vi "LoadApplicationConfig.vi"(8 "error in (no error)":errorcluster) -> (0 "error out":errorcluster, 2 "Config Cluster":T1, 3 "refnum out":T7)   [LabVIEW 2026]
uses:
  <vilib>/Utility/config.llb/Config Data RefNum.ctl
  Controls/Vibration_Monitor_Config.ctl
  Controls/Vibration_Profile.ctl
  Controls/System_Settings.ctl
  Controls/Options.ctl
  Controls/Relay_Profile.ctl
  Controls/RPM_Profile.ctl
  <vilib>/Utility/config.llb/Read Key (String).vi
  <vilib>/Utility/config.llb/Read Key (I32).vi
  <vilib>/Utility/config.llb/Read Key (Double).vi
  <vilib>/Utility/config.llb/NI_LVConfig.lvlib
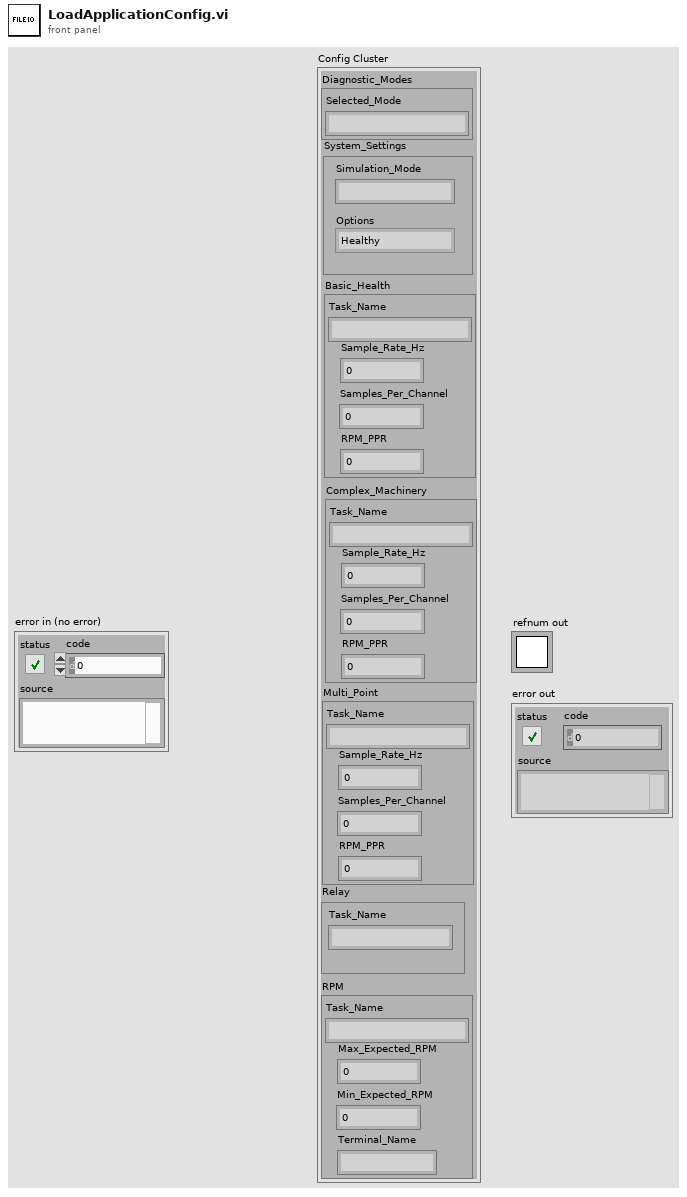
[diagram p1: front panel]
types:
  T1 = typedef "Vibration_Monitor_Config.ctl" = cluster{"Diagnostic_Modes":cluster{"Selected_Mode":string}, "Basic_Health":T2, "Complex_Machinery":T2, "Multi_Point":T2, "System_Settings":T3, "Relay":T5, "RPM":T6}
  T2 = typedef "Vibration_Profile.ctl" = cluster{"Task_Name":string, "Sample_Rate_Hz":dbl, "Samples_Per_Channel":i32, "RPM_PPR ":dbl}
  T3 = typedef "System_Settings.ctl" = cluster{"Simulation_Mode ":string, "Options":T4}
  T4 = typedef "Options.ctl" = enum16{"Healthy", "Unbalance_Alert", "Bearing_Fault_Critical", "Sweep_Test"}
  T5 = typedef "Relay_Profile.ctl" = cluster{"Task_Name":string}
  T6 = typedef "RPM_Profile.ctl" = cluster{"Task_Name":string, "Max_Expected_RPM":dbl, "Min_Expected_RPM":dbl, "Terminal_Name":string}
  T7 = typedef "NI_LVConfig.lvlib/Config Data RefNum.ctl" = refnum<k1>
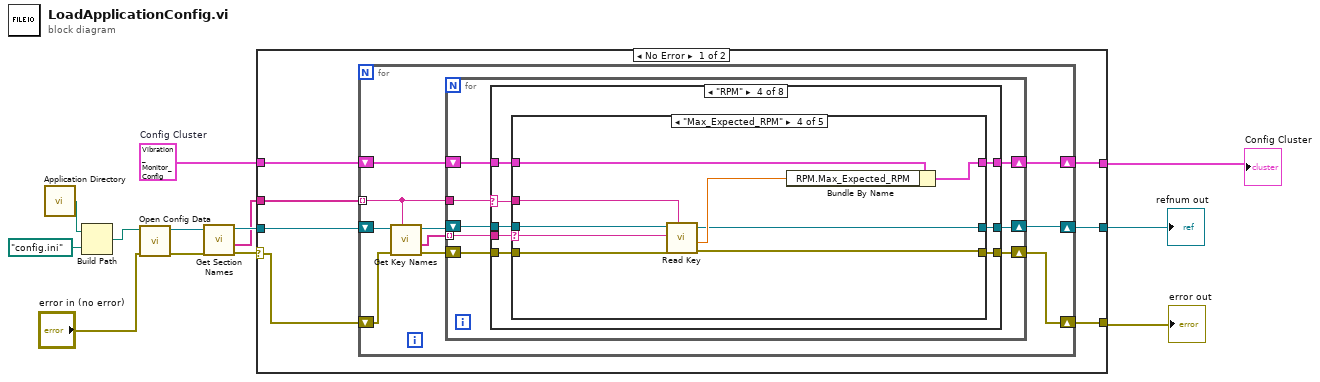
[diagram p0: block diagram]
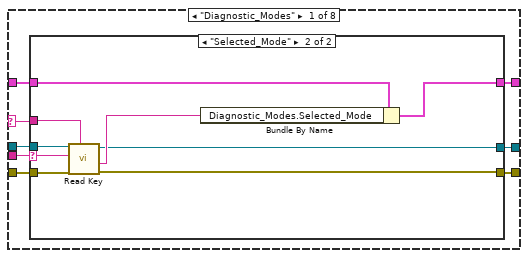
[diagram p2: hidden frame]
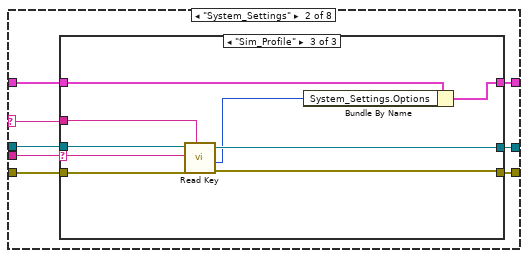
[diagram p4: hidden frame]
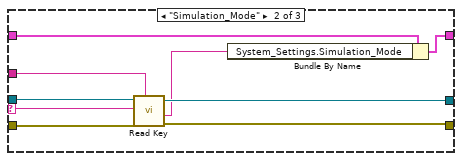
[diagram p6: hidden frame]
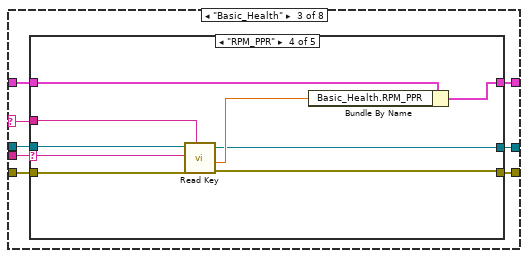
[diagram p7: hidden frame]
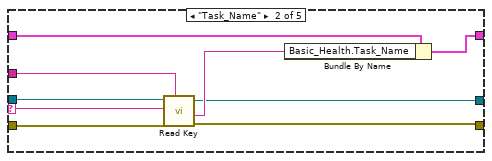
[diagram p9: hidden frame]
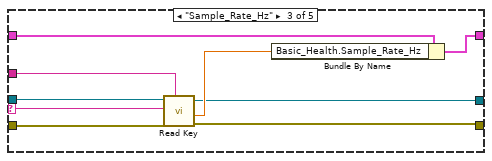
[diagram p10: hidden frame]
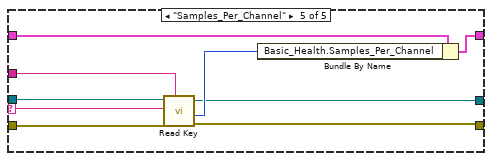
[diagram p11: hidden frame]
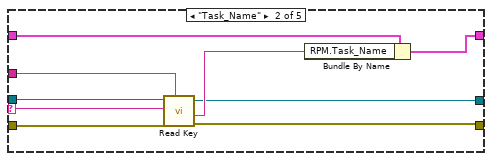
[diagram p13: hidden frame]
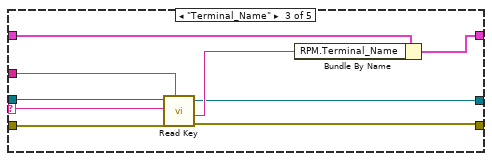
[diagram p14: hidden frame]
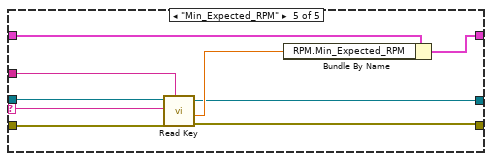
[diagram p15: hidden frame]
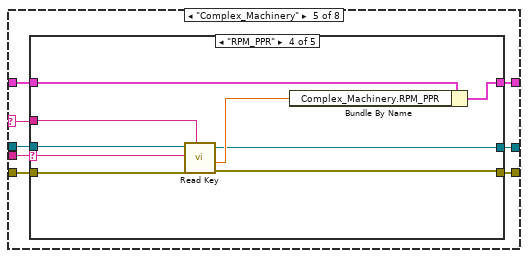
[diagram p16: hidden frame]
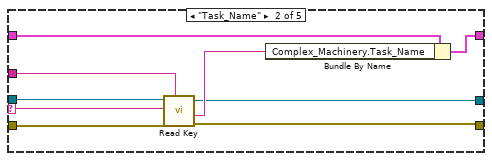
[diagram p18: hidden frame]
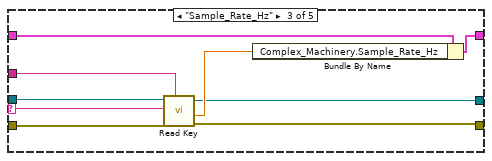
[diagram p19: hidden frame]
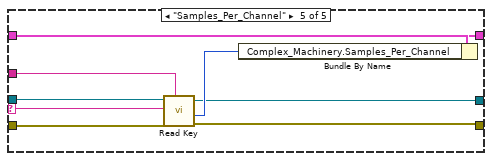
[diagram p20: hidden frame]
diagram:
  w2 = T1 {"Diagnostic_Modes"={"Selected_Mode"=""}, "Basic_Health"={"Task_Name"="", "Sample_Rate_Hz"=0.0, "Samples_Per_Channel"=0, "RPM_PPR "=0.0}, "Complex_Machinery"={"Task_Name"="", "Sample_Rate_Hz"=0.0, "Samples_Per_Channel"=0, "RPM_PPR "=0.0}, "Multi_Point"={"Task_Name"="", "Sample_Rate_Hz"=0.0, "Samples_Per_Channel"=0, "RPM_PPR "=0.0}, "System_Settings"={"Simulation_Mode "="", "Options"=enum."Healthy"}, "Relay"={"Task_Name"=""}, "RPM"={"Task_Name"="", "Max_Expected_RPM"=0.0, "Min_Expected_RPM"=0.0, "Terminal_Name"=""}}  # Config Cluster
  n1 = call <vilib>:"Application Directory.vi"() -> ("Application Directory"=w12:path)
  n2 = Build Path(base path=w12, name or relative path=path "config.ini") -> (appended path=w13:path)
  n3 = call <vilib>:"Open Config Data.vi"("error in (no error)"="error in (no error)", "configuration file path"=w13) -> ("error out"=w9:errorcluster, "refnum"=w10:T7)  [unwired: 7 in, 1 out]
  n4 = call <vilib>:"Get Section Names.vi"("error in (no error)"=w9, "refnum"=w10) -> ("error out"=w6:errorcluster, "section names"=w4:string[], "refnum out"=w5:T7)  [unwired: 7 in]
  n5 = case shown="No Error" w6 {
    selector: w6 -> [w19 w319]
    tunnel: [w17 w319] -> w8
    tunnel: w5 -> [w20 w318]
    tunnel: w4 -> [w18 _]
    tunnel: [w16 w318] -> w3
    tunnel: w2 -> [w15 w317]
    tunnel: [w14 w317] -> w1
    frame No Error {
      n6 = for {
        tunnel: w18 -> [w21] mode=indexing
        shift-right: [w26] -> w17
        shift-left: w19 -> [w29]
        shift-right: [w24] -> w16
        shift-left: w20 -> [w30]
        shift-right: [w22] -> w14
        shift-left: w15 -> [w23]
        n7 = call <vilib>:"Get Key Names.vi"("section"=w21, "error in (no error)"=w29, "refnum"=w30) -> ("error out"=w28:errorcluster, "key names"=w25:string[], "refnum out"=w27:T7)  [unwired: 5 in, 1 out]
        n8 = for {
          shift-right: [w33] -> w26
          shift-left: w28 -> [w35]
          tunnel: w25 -> [w36] mode=indexing
          shift-right: [w32] -> w24
          shift-left: w27 -> [w34]
          shift-right: [w38] -> w22
          shift-left: w23 -> [w37]
          tunnel: w21 -> [w31]
          n9 = case shown="\"RPM\"" w31 {
            selector: w31 -> [w39 w59 w88 w135 w182 w229 w276 _]
            tunnel: [w46 w66 w95 w142 w189 w236 w283 w316] -> w38
            tunnel: w37 -> [w45 w65 w94 w141 w188 w235 w282 w316]
            tunnel: w36 -> [w44 w64 w93 w140 w187 w234 w281 _]
            tunnel: w35 -> [w43 w63 w92 w139 w186 w233 w280 w314]
            tunnel: w34 -> [w42 w62 w91 w138 w185 w232 w279 w315]
            tunnel: [w41 w61 w90 w137 w184 w231 w278 w314] -> w33
            tunnel: [w40 w60 w89 w136 w183 w230 w277 w315] -> w32
            frame "Diagnostic_Modes" {
              n10 = case shown="\"Selected_Mode\"" w44 {
                selector: w44 -> [_ w57]
                tunnel: [w49 w56] -> w46
                tunnel: w45 -> [w49 w58]
                tunnel: w39 -> [_ w55]
                tunnel: w43 -> [w48 w53]
                tunnel: w42 -> [w47 w52]
                tunnel: [w48 w51] -> w41
                tunnel: [w47 w50] -> w40
                frame Default {
                }
                frame "Selected_Mode" {
                  n11 = call-poly <vilib>:"Read Key.vi"("section"=w55, "error in (no error)"=w53, "key"=w57, "refnum"=w52) -> ("error out"=w51:errorcluster, "value"=w54:string, "refnum out"=w50:T7)  [unwired: 4 in, 1 out]
                  n12 = Bundle By Name(cluster=w58, "Diagnostic_Modes.Selected_Mode"=w54) -> (w56:T1)
                }
              }
            }
            frame "System_Settings" {
              n13 = case shown="\"Sim_Profile\"" w64 {
                selector: w64 -> [_ w73 w82]
                tunnel: [w69 w77 w86] -> w66
                tunnel: w65 -> [w69 w78 w87]
                tunnel: w59 -> [_ w74 w83]
                tunnel: w63 -> [w67 w75 w84]
                tunnel: w62 -> [w68 w76 w85]
                tunnel: [w67 w72 w81] -> w61
                tunnel: [w68 w71 w80] -> w60
                frame Default {
                }
                frame "Simulation_Mode" {
                  n14 = call-poly <vilib>:"Read Key.vi"("section"=w74, "error in (no error)"=w75, "key"=w73, "refnum"=w76) -> ("error out"=w72:errorcluster, "value"=w70:string, "refnum out"=w71:T7)  [unwired: 4 in, 1 out]
                  n15 = Bundle By Name(cluster=w78, "System_Settings.Simulation_Mode"=w70) -> (w77:T1)
                }
                frame "Sim_Profile" {
                  n16 = call-poly <vilib>:"Read Key.vi"("section"=w83, "error in (no error)"=w84, "key"=w82, "refnum"=w85) -> ("error out"=w81:errorcluster, "value"=w79:i32, "refnum out"=w80:T7)  [unwired: 4 in, 1 out]
                  n17 = Bundle By Name(cluster=w87, "System_Settings.Options"=w79) -> (w86:T1)
                }
              }
            }
            frame "Basic_Health" {
              n18 = case shown="\"RPM_PPR\"" w93 {
                selector: w93 -> [_ w101 w110 w119 w128]
                tunnel: [w98 w106 w115 w124 w133] -> w95
                tunnel: w94 -> [w98 w107 w116 w125 w134]
                tunnel: w88 -> [_ w103 w112 w121 w130]
                tunnel: w92 -> [w96 w104 w113 w122 w131]
                tunnel: w91 -> [w97 w105 w114 w123 w132]
                tunnel: [w96 w100 w109 w118 w127] -> w90
                tunnel: [w97 w99 w108 w117 w126] -> w89
                frame Default {
                }
                frame "Task_Name" {
                  n19 = call-poly <vilib>:"Read Key.vi"("section"=w103, "error in (no error)"=w104, "key"=w101, "refnum"=w105) -> ("error out"=w100:errorcluster, "value"=w102:string, "refnum out"=w99:T7)  [unwired: 4 in, 1 out]
                  n20 = Bundle By Name(cluster=w107, "Basic_Health.Task_Name"=w102) -> (w106:T1)
                }
                frame "Sample_Rate_Hz" {
                  n21 = call-poly <vilib>:"Read Key.vi"("section"=w112, "error in (no error)"=w113, "key"=w110, "refnum"=w114) -> ("error out"=w109:errorcluster, "value"=w111:dbl, "refnum out"=w108:T7)  [unwired: 4 in, 1 out]
                  n22 = Bundle By Name(cluster=w116, "Basic_Health.Sample_Rate_Hz"=w111) -> (w115:T1)
                }
                frame "RPM_PPR" {
                  n23 = call-poly <vilib>:"Read Key.vi"("section"=w121, "error in (no error)"=w122, "key"=w119, "refnum"=w123) -> ("error out"=w118:errorcluster, "value"=w120:dbl, "refnum out"=w117:T7)  [unwired: 4 in, 1 out]
                  n24 = Bundle By Name(cluster=w125, "Basic_Health.RPM_PPR"=w120) -> (w124:T1)
                }
                frame "Samples_Per_Channel" {
                  n25 = call-poly <vilib>:"Read Key.vi"("section"=w130, "error in (no error)"=w131, "key"=w128, "refnum"=w132) -> ("error out"=w127:errorcluster, "value"=w129:i32, "refnum out"=w126:T7)  [unwired: 4 in, 1 out]
                  n26 = Bundle By Name(cluster=w134, "Basic_Health.Samples_Per_Channel"=w129) -> (w133:T1)
                }
              }
            }
            frame "RPM" {
              n27 = case shown="\"Max_Expected_RPM\"" w140 {
                selector: w140 -> [_ w148 w157 w166 w175]
                tunnel: [w145 w153 w162 w171 w180] -> w142
                tunnel: w141 -> [w145 w154 w163 w172 w181]
                tunnel: w135 -> [_ w150 w159 w168 w177]
                tunnel: w139 -> [w143 w151 w160 w169 w178]
                tunnel: w138 -> [w144 w152 w161 w170 w179]
                tunnel: [w143 w147 w156 w165 w174] -> w137
                tunnel: [w144 w146 w155 w164 w173] -> w136
                frame Default {
                }
                frame "Task_Name" {
                  n28 = call-poly <vilib>:"Read Key.vi"("section"=w150, "error in (no error)"=w151, "key"=w148, "refnum"=w152) -> ("error out"=w147:errorcluster, "value"=w149:string, "refnum out"=w146:T7)  [unwired: 4 in, 1 out]
                  n29 = Bundle By Name(cluster=w154, "RPM.Task_Name"=w149) -> (w153:T1)
                }
                frame "Terminal_Name" {
                  n30 = call-poly <vilib>:"Read Key.vi"("section"=w159, "error in (no error)"=w160, "key"=w157, "refnum"=w161) -> ("error out"=w156:errorcluster, "value"=w158:string, "refnum out"=w155:T7)  [unwired: 4 in, 1 out]
                  n31 = Bundle By Name(cluster=w163, "RPM.Terminal_Name"=w158) -> (w162:T1)
                }
                frame "Max_Expected_RPM" {
                  n32 = call-poly <vilib>:"Read Key.vi"("section"=w168, "error in (no error)"=w169, "key"=w166, "refnum"=w170) -> ("error out"=w165:errorcluster, "value"=w167:dbl, "refnum out"=w164:T7)  [unwired: 4 in, 1 out]
                  n33 = Bundle By Name(cluster=w172, "RPM.Max_Expected_RPM"=w167) -> (w171:T1)
                }
                frame "Min_Expected_RPM" {
                  n34 = call-poly <vilib>:"Read Key.vi"("section"=w177, "error in (no error)"=w178, "key"=w175, "refnum"=w179) -> ("error out"=w174:errorcluster, "value"=w176:dbl, "refnum out"=w173:T7)  [unwired: 4 in, 1 out]
                  n35 = Bundle By Name(cluster=w181, "RPM.Min_Expected_RPM"=w176) -> (w180:T1)
                }
              }
            }
            frame "Complex_Machinery" {
              n36 = case shown="\"RPM_PPR\"" w187 {
                selector: w187 -> [_ w195 w204 w213 w222]
                tunnel: [w192 w200 w209 w218 w227] -> w189
                tunnel: w188 -> [w192 w201 w210 w219 w228]
                tunnel: w182 -> [_ w197 w206 w215 w224]
                tunnel: w186 -> [w190 w198 w207 w216 w225]
                tunnel: w185 -> [w191 w199 w208 w217 w226]
                tunnel: [w190 w194 w203 w212 w221] -> w184
                tunnel: [w191 w193 w202 w211 w220] -> w183
                frame Default {
                }
                frame "Task_Name" {
                  n37 = call-poly <vilib>:"Read Key.vi"("section"=w197, "error in (no error)"=w198, "key"=w195, "refnum"=w199) -> ("error out"=w194:errorcluster, "value"=w196:string, "refnum out"=w193:T7)  [unwired: 4 in, 1 out]
                  n38 = Bundle By Name(cluster=w201, "Complex_Machinery.Task_Name"=w196) -> (w200:T1)
                }
                frame "Sample_Rate_Hz" {
                  n39 = call-poly <vilib>:"Read Key.vi"("section"=w206, "error in (no error)"=w207, "key"=w204, "refnum"=w208) -> ("error out"=w203:errorcluster, "value"=w205:dbl, "refnum out"=w202:T7)  [unwired: 4 in, 1 out]
                  n40 = Bundle By Name(cluster=w210, "Complex_Machinery.Sample_Rate_Hz"=w205) -> (w209:T1)
                }
                frame "RPM_PPR" {
                  n41 = call-poly <vilib>:"Read Key.vi"("section"=w215, "error in (no error)"=w216, "key"=w213, "refnum"=w217) -> ("error out"=w212:errorcluster, "value"=w214:dbl, "refnum out"=w211:T7)  [unwired: 4 in, 1 out]
                  n42 = Bundle By Name(cluster=w219, "Complex_Machinery.RPM_PPR"=w214) -> (w218:T1)
                }
                frame "Samples_Per_Channel" {
                  n43 = call-poly <vilib>:"Read Key.vi"("section"=w224, "error in (no error)"=w225, "key"=w222, "refnum"=w226) -> ("error out"=w221:errorcluster, "value"=w223:i32, "refnum out"=w220:T7)  [unwired: 4 in, 1 out]
                  n44 = Bundle By Name(cluster=w228, "Complex_Machinery.Samples_Per_Channel"=w223) -> (w227:T1)
                }
              }
            }
            frame "Multi_Point" {
              n45 = case shown="\"RPM_PPR\"" w234 {
                selector: w234 -> [_ w242 w251 w260 w269]
                tunnel: [w239 w247 w256 w265 w274] -> w236
                tunnel: w235 -> [w239 w248 w257 w266 w275]
                tunnel: w229 -> [_ w244 w253 w262 w271]
                tunnel: w233 -> [w237 w245 w254 w263 w272]
                tunnel: w232 -> [w238 w246 w255 w264 w273]
                tunnel: [w237 w241 w250 w259 w268] -> w231
                tunnel: [w238 w240 w249 w258 w267] -> w230
                frame Default {
                }
                frame "Task_Name" {
                  n46 = call-poly <vilib>:"Read Key.vi"("section"=w244, "error in (no error)"=w245, "key"=w242, "refnum"=w246) -> ("error out"=w241:errorcluster, "value"=w243:string, "refnum out"=w240:T7)  [unwired: 4 in, 1 out]
                  n47 = Bundle By Name(cluster=w248, "Multi_Point.Task_Name"=w243) -> (w247:T1)
                }
                frame "Sample_Rate_Hz" {
                  n48 = call-poly <vilib>:"Read Key.vi"("section"=w253, "error in (no error)"=w254, "key"=w251, "refnum"=w255) -> ("error out"=w250:errorcluster, "value"=w252:dbl, "refnum out"=w249:T7)  [unwired: 4 in, 1 out]
                  n49 = Bundle By Name(cluster=w257, "Multi_Point.Sample_Rate_Hz"=w252) -> (w256:T1)
                }
                frame "RPM_PPR" {
                  n50 = call-poly <vilib>:"Read Key.vi"("section"=w262, "error in (no error)"=w263, "key"=w260, "refnum"=w264) -> ("error out"=w259:errorcluster, "value"=w261:dbl, "refnum out"=w258:T7)  [unwired: 4 in, 1 out]
                  n51 = Bundle By Name(cluster=w266, "Multi_Point.RPM_PPR"=w261) -> (w265:T1)
                }
                frame "Samples_Per_Channel" {
                  n52 = call-poly <vilib>:"Read Key.vi"("section"=w271, "error in (no error)"=w272, "key"=w269, "refnum"=w273) -> ("error out"=w268:errorcluster, "value"=w270:i32, "refnum out"=w267:T7)  [unwired: 4 in, 1 out]
                  n53 = Bundle By Name(cluster=w275, "Multi_Point.Samples_Per_Channel"=w270) -> (w274:T1)
                }
              }
            }
            frame "Relay" {
              n54 = case shown="\"Task_Name\"" w281 {
                selector: w281 -> [_ w289 w298 w307]
                tunnel: [w286 w294 w303 w312] -> w283
                tunnel: w282 -> [w286 w295 w304 w313]
                tunnel: w276 -> [_ w291 w300 w309]
                tunnel: w280 -> [w284 w292 w301 w310]
                tunnel: w279 -> [w285 w293 w302 w311]
                tunnel: [w284 w288 w297 w306] -> w278
                tunnel: [w285 w287 w296 w305] -> w277
                frame Default {
                }
                frame "Task_Name" {
                  n55 = call-poly <vilib>:"Read Key.vi"("section"=w291, "error in (no error)"=w292, "key"=w289, "refnum"=w293) -> ("error out"=w288:errorcluster, "value"=w290:string, "refnum out"=w287:T7)  [unwired: 4 in, 1 out]
                  n56 = Bundle By Name(cluster=w295, "Relay.Task_Name"=w290) -> (w294:T1)
                }
                frame "Sample_Rate_Hz" {
                  n57 = call-poly <vilib>:"Read Key.vi"("section"=w300, "error in (no error)"=w301, "key"=w298, "refnum"=w302) -> ("error out"=w297:errorcluster, "value"=w299:dbl, "refnum out"=w296:T7)  [unwired: 4 in, 1 out]
                  n58 = Bundle By Name(cluster=w304, "Multi_Point.Sample_Rate_Hz"=w299) -> (w303:T1)
                }
                frame "Samples_Per_Channel" {
                  n59 = call-poly <vilib>:"Read Key.vi"("section"=w309, "error in (no error)"=w310, "key"=w307, "refnum"=w311) -> ("error out"=w306:errorcluster, "value"=w308:i32, "refnum out"=w305:T7)  [unwired: 4 in, 1 out]
                  n60 = Bundle By Name(cluster=w313, "Multi_Point.Samples_Per_Channel"=w308) -> (w312:T1)
                }
              }
            }
            frame Default {
            }
          }
        }
      }
    }
    frame Error {
    }
  }
  "error out" <- w8
  "refnum out" <- w3
  "Config Cluster" <- w1
